vi "Distance Drive PID.vi"(4 "reinitialize? (F)":bool, 5 "output range":T1, 6 "PID Params":T2, 7 "Setpoint":dbl, 8 "Max Stop Speed":dbl, 9 "Distance Stop":dbl, 10 "Current Speed":dbl, 11 "Current Distance":dbl) -> (0 "Finished":bool, 2 "output":dbl)   [LabVIEW 2015]
uses:
  Common Code/Drivetrain Output Range.ctl
  <vilib>/addons/control/pid/pid.llb/PID (DBL).vi
  <vilib>/addons/control/pid/NI_PID_pid.lvlib
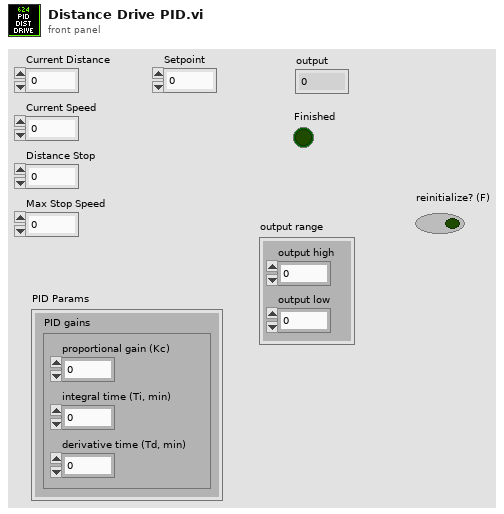
[diagram p1: front panel]
types:
  T1 = typedef "Drivetrain Output Range.ctl" = cluster{"output high":dbl, "output low":dbl}
  T2 = cluster{"PID gains":cluster{"proportional gain (Kc)":dbl, "integral time (Ti, min)":dbl, "derivative time (Td, min)":dbl}}
  T3 = cluster{"proportional gain (Kc)":dbl, "integral time (Ti, min)":dbl, "derivative time (Td, min)":dbl}
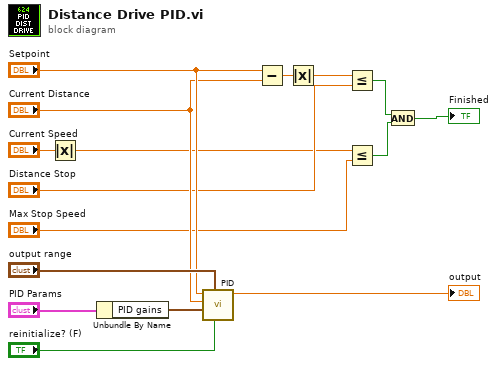
[diagram p0: block diagram]
diagram:
  n1 = Absolute Value(x="Current Speed") -> (abs(x)=w4:dbl)
  n2 = Unbundle By Name("PID Params") -> ("PID gains"=w14:T3)
  n3 = call-poly <vilib>:"PID.vi"("reinitialize? (F)"="reinitialize? (F)", "output range"="output range", "PID gains"=w14, "process variable"="Current Distance", "setpoint"="Setpoint") -> ("output"=→"output":dbl)  [unwired: 5 in, 1 out]
  n4 = Subtract(x="Setpoint", y="Current Distance") -> (x-y=w9:dbl)
  n5 = Absolute Value(x=w9) -> (abs(x)=w7:dbl)
  n6 = Less Or Equal?(x=w7, y="Distance Stop") -> (x <= y?=w3:bool)
  n7 = Less Or Equal?(x=w4, y="Max Stop Speed") -> (x <= y?=w2:bool)
  n8 = And(x=w3, y=w2) -> (x .and. y?=→"Finished":bool)
